vi "VNA_measure.vi"(8 "error in (no error)":errorcluster, 10 "timeout":dbl, 11 "Resource Name In":refnum<k15>) -> (0 "error out":errorcluster, 3 "Resource Name Out":refnum<k15>)   [LabVIEW 2017]
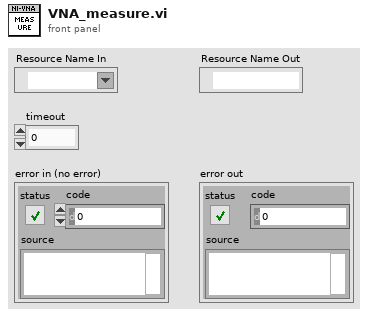
[diagram p1: front panel]
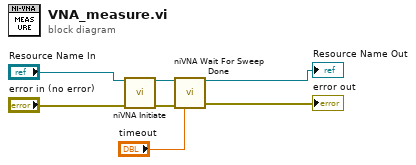
[diagram p0: block diagram]
diagram:
  n1 = call <instrlib>:"niVNA Initiate.vi"("instrument handle"="Resource Name In", "error in"="error in (no error)") -> ("instrument handle out"=w3:refnum<k15>, "error out"=w4:errorcluster)  [unwired: 12 in]
  n2 = call <instrlib>:"niVNA Wait For Sweep Done.vi"("instrument handle"=w3, "error in"=w4, "timeout"="timeout") -> ("instrument handle out"=→"Resource Name Out":refnum<k15>, "error out"=→"error out":errorcluster)  [unwired: 11 in]
